vi "Injector global.vi"() -> ()   [LabVIEW 2016]
panel:
  out "Convert":bool
  in  "Rare  field":dbl
  in  "Stable field":dbl
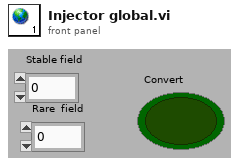
[diagram p1: front panel]
diagram:
